vi "XYZ stage handler_MD.vi"   [LabVIEW 2012]
uses:
  <vilib>/Analysis/coordinate.llb/Euler Rotation Order.ctl
  GFG/GFGfpRefGet.vi
  GFG/GFGbooleanGet.vi
  GFG/GFGnumericGet.vi
  <vilib>/Analysis/coordinate.llb/3D Cartesian Coordinate Rotation (Euler) (Scalar).vi
  GFG/GFG library.lvlib
  <vilib>/Utility/VariantDataType/Type.ctl
  <vilib>/Utility/VariantDataType/VariantType.lvlib
  <vilib>/Analysis/NI_AALPro.lvlib
types:
  T1 = enum16{"none", "quit", "Press", "Long Press", "Long Press finished", "Short Press finished"}
  T2 = cluster{"WaveformChartRef":refnum<vi>, "DigitalRef":refnum<vi>, "ArrayRef":refnum<vi>, "TabControlRef":refnum<vi>, "EnumRef":refnum<vi>, "RingRef":refnum<vi>, "BooleanRef":refnum<vi>, "KnobRef":refnum<vi>, "SlideRef":refnum<vi>, "PathRef":refnum<vi>, "StringRef":refnum<vi>, "ComboBox":refnum<vi>, "WaveformGraphRef":refnum<vi>}
  T3 = cluster{"moveXabs":dbl, "moveYabs":dbl, "moveZabs":dbl}
  T4 = typedef "NI_AALPro.lvlib/Euler Rotation Order.ctl" = u16
  T5 = cluster{"Numeric":dbl, "Numeric":dbl, "Numeric":dbl}
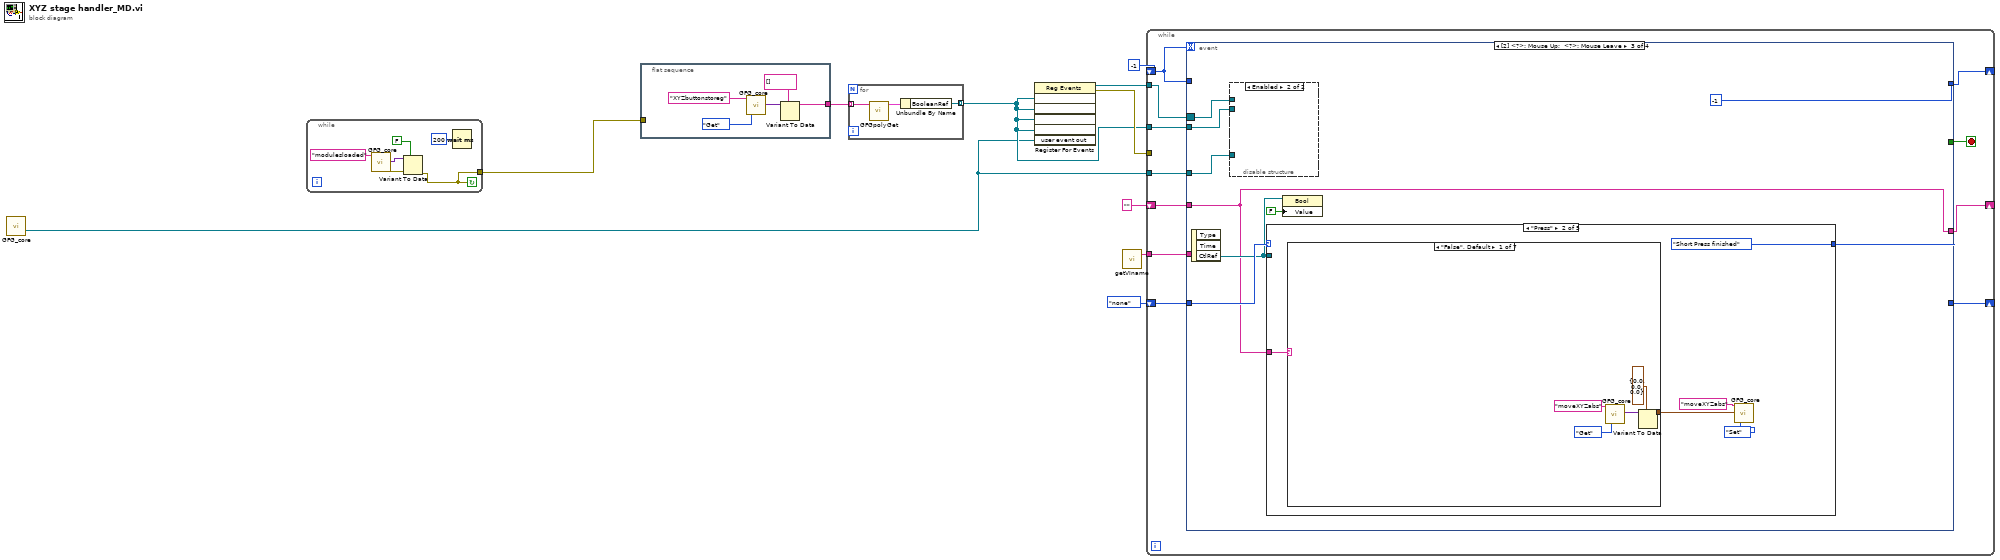
[diagram p0: block diagram]
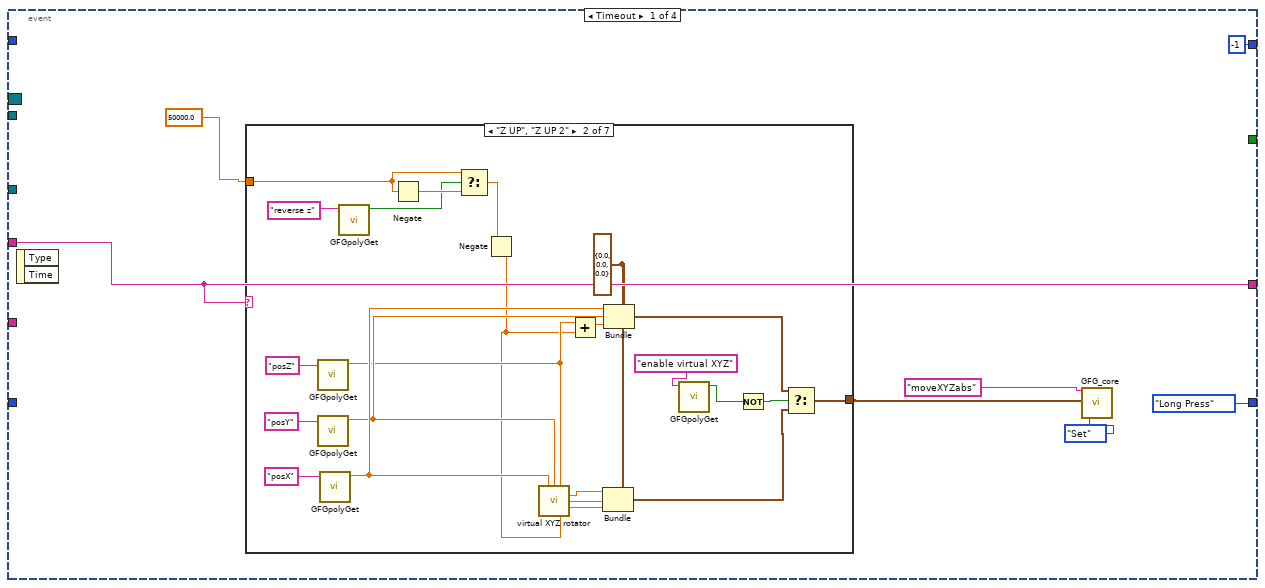
[diagram p2: hidden frame]
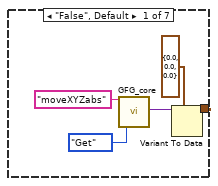
[diagram p3: hidden frame]
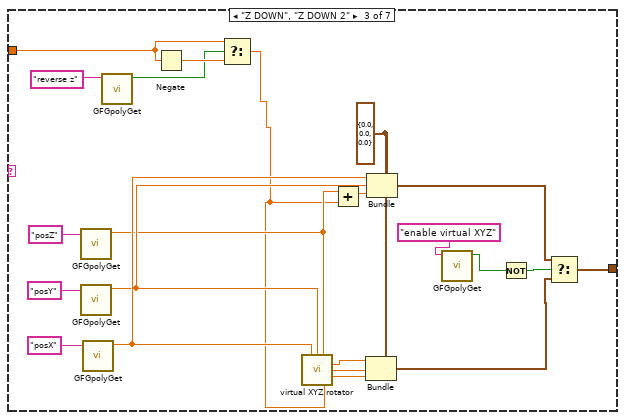
[diagram p4: hidden frame]
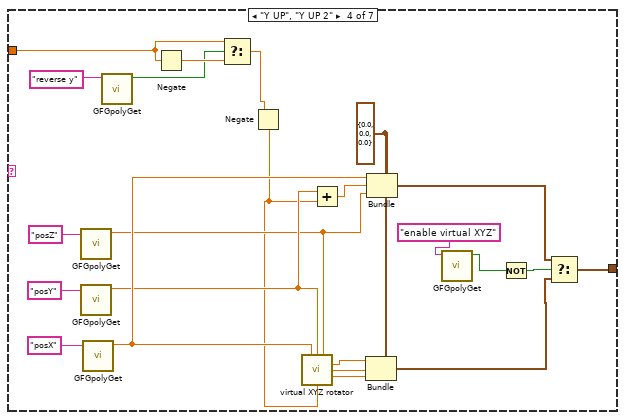
[diagram p5: hidden frame]
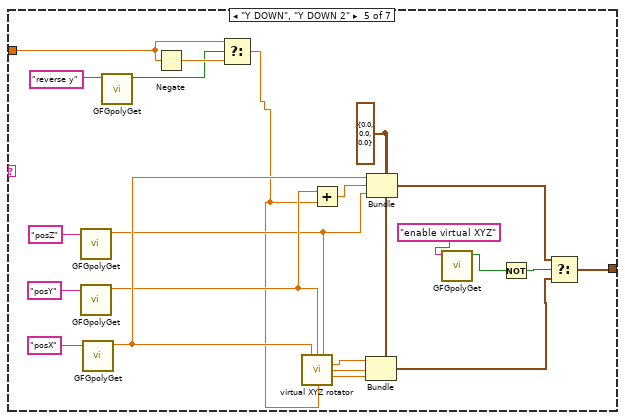
[diagram p6: hidden frame]
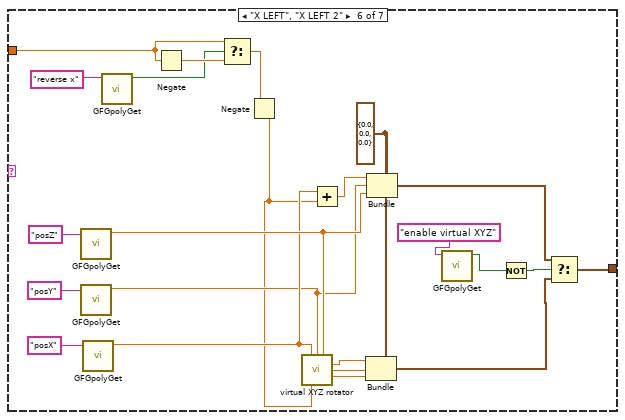
[diagram p7: hidden frame]
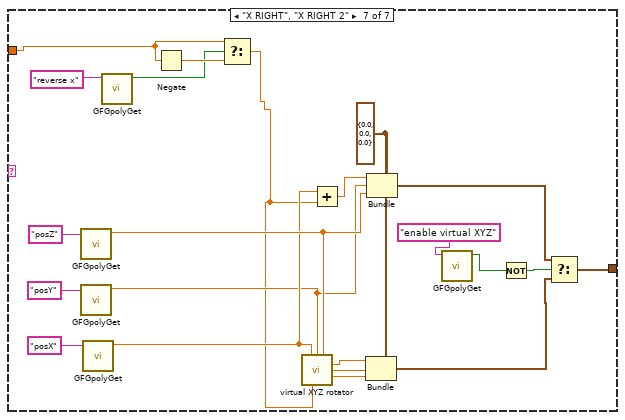
[diagram p8: hidden frame]
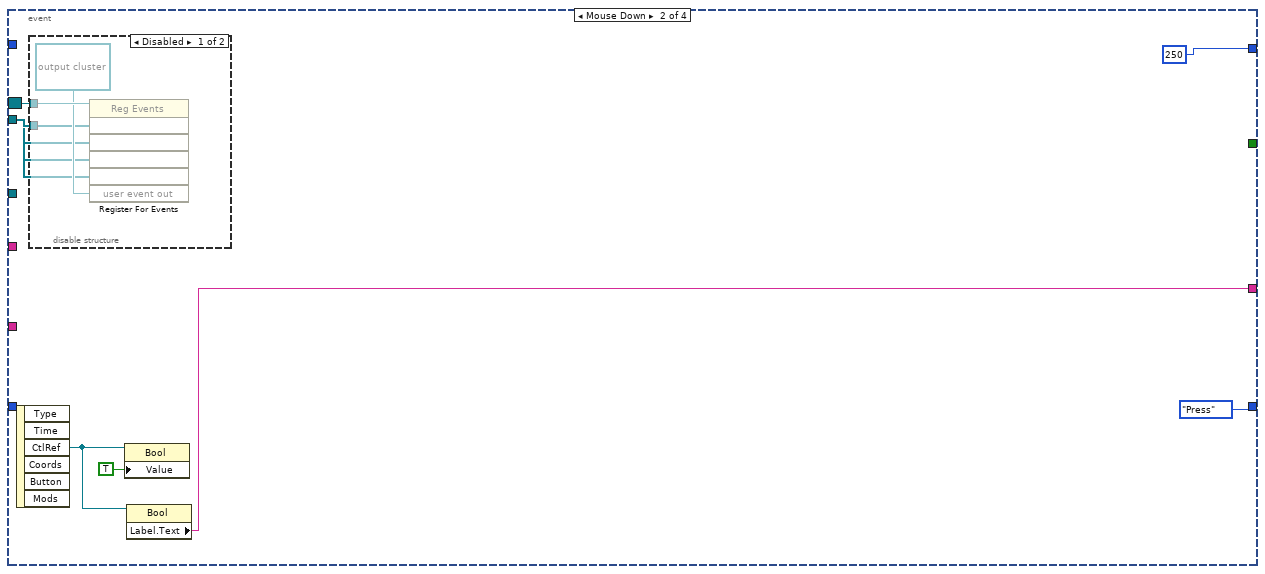
[diagram p9: hidden frame]
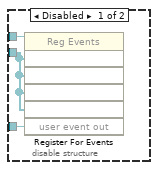
[diagram p11: hidden frame]
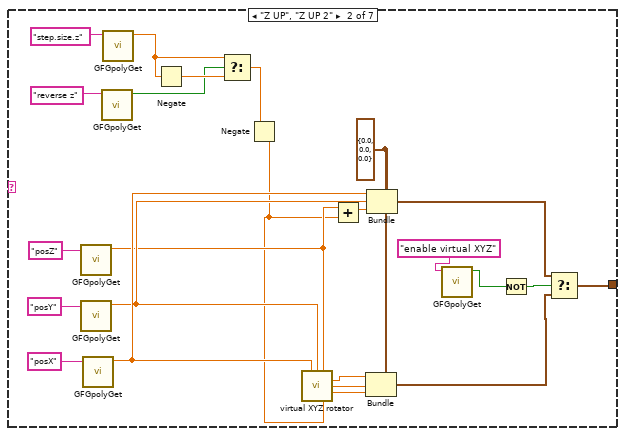
[diagram p13: hidden frame]
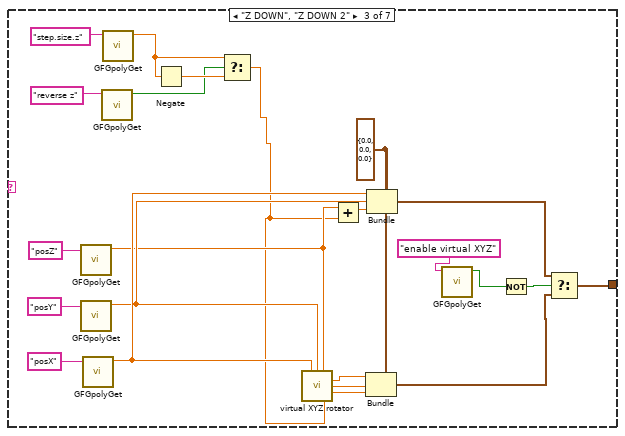
[diagram p14: hidden frame]
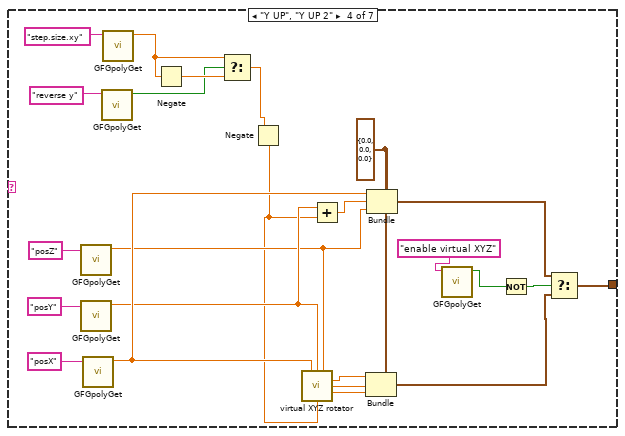
[diagram p15: hidden frame]
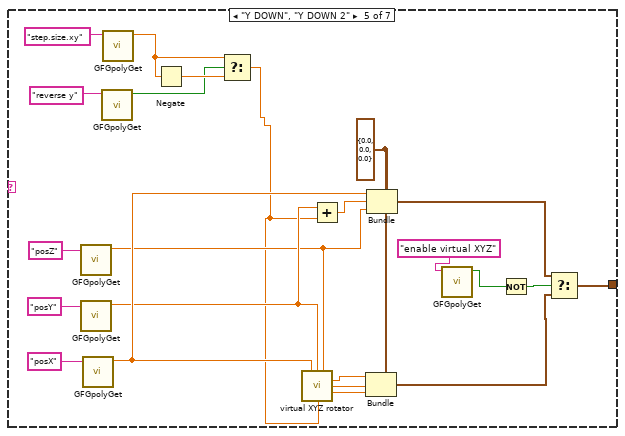
[diagram p16: hidden frame]
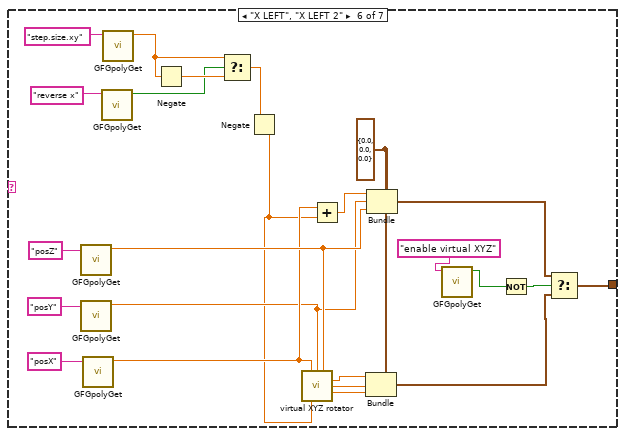
[diagram p17: hidden frame]
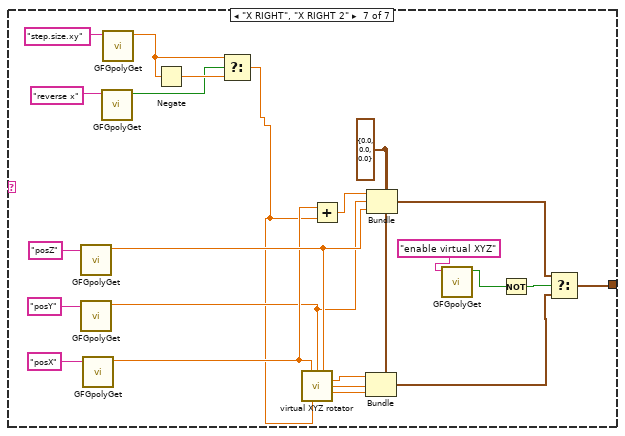
[diagram p18: hidden frame]
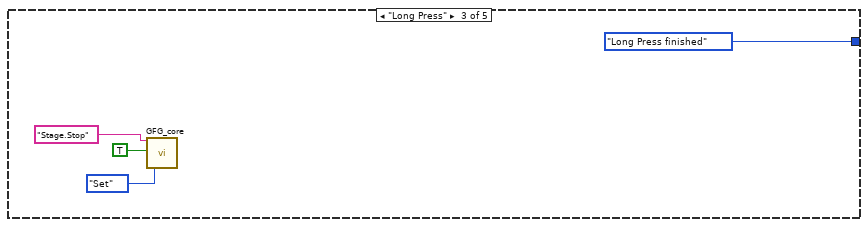
[diagram p19: hidden frame]
diagram:
  n1 = call "GFG_core.vi"() -> ("user event out"=w2:refnum<user-event>)  [unwired: 13 in, 6 out]
  n2 = while {
    tunnel: [w11] -> w1
    stop <- w11 continue-if-true
    n3 = call "GFG_core.vi"("Variable Name in"="modulesloaded") -> ("Variant Out"=w12:variant, "error out"=w14:errorcluster)  [unwired: 12 in, 5 out]
    n4 = Variant To Data(error in=w14, type=FALSE, Variant=w12) -> (error out=w11:errorcluster)  [unwired: 1 out]
    n5 = Wait (ms)(milliseconds to wait=u32 200) -> ()  [unwired: 1 out]
  }
  n6 = flat-sequence {
    tunnel: [w21] -> w3
    tunnel: w1 -> [_]
    frame #0 {
      n7 = call "GFG_core.vi"("Variable Name in"="XYZbuttonstoreg", "Action"=enum16{"Init", "Set", "Get"}."Get") -> ("Variant Out"=w17:variant)  [unwired: 11 in, 6 out]
      n8 = Variant To Data(type=string[] [], Variant=w17) -> (data=w21:string[])  [unwired: 1 in, 1 out]
    }
  }
  n9 = for {
    tunnel: w3 -> [w23] mode=indexing
    tunnel: [w22] -> w5 mode=indexing
    n10 = call-poly "GFGpolyGet.vi"("Variable Name in"=w23) -> ("output cluster"=w24:T2)  [unwired: 9 in, 1 out]
    n11 = Unbundle By Name(w24) -> ("BooleanRef"=w22:refnum<vi>)
  }
  n12 = register-events(w5, w5, w5, w5, w2) -> (reference out=w4:refnum<event-registration>, error out=w6:errorcluster)  [unwired: 2 in]
  n13 = call "getVIname.vi"() -> ("VI name"=w7:string)  [unwired: 19 in]
  n14 = while {
    shift-right: [w33] -> _
    shift-left: -1 -> [w34]
    shift-right: [w31] -> _
    shift-left: T1."none" ("Enum") -> [w32]
    shift-right: [w30] -> _
    shift-left: "" ("Label.Text") -> [w29]
    tunnel: w5 -> [w28]
    tunnel: w2 -> [w27]
    tunnel: w4 -> [w26]
    tunnel: w7 -> [w25]
    tunnel: w6 -> [_]
    stop <- w35 stop-if-true
    n15 = event shown="[2] <?>: Mouse Up;  <?>: Mouse Leave" {
      selector: w26 -> [_ w186 w195 _]
      dyn-events: _ -> [_ _ _ _]
      timeout: w34 -> [_ _ _ _]
      tunnel: [_ _ _ w375] -> w35
      tunnel: w34 -> [_ _ _ w365]
      tunnel: [-1 250 -1 w364] -> w33
      tunnel: w32 -> [_ _ w200 w374]
      tunnel: [T1."Long Press" ("Enum") T1."Press" ("Enum") w199 w374] -> w31
      tunnel: [w40 w187 w193 w371] -> w30
      tunnel: w29 -> [w40 _ w193 w371]
      tunnel: w28 -> [_ w183 w194 _]
      tunnel: w27 -> [_ _ w196 _]
      tunnel: w25 -> [_ _ _ w372]
      event Timeout {
        n16 = event-data() -> ()  [unwired: 1 in, 2 out]
        n17 = case shown="\"Z UP\", \"Z UP 2\"" w40 {
          tunnel: [w43 w53 w75 w101 w123 w147 w169] -> w36
          tunnel: 50000.0 ("-x") -> [_ w48 w71 w93 w116 w138 w161]
          frame "False", Default {
            n18 = call "GFG_core.vi"("Variable Name in"="moveXYZabs", "Action"=enum16{"Init", "Set", "Get"}."Get") -> ("Variant Out"=w45:variant)  [unwired: 11 in, 6 out]
            n19 = Variant To Data(type=T3 {"moveXabs"=0.0, "moveYabs"=0.0, "moveZabs"=0.0} ("output cluster"), Variant=w45) -> (data=w43:T3)  [unwired: 1 in, 1 out]
          }
          frame "Z UP", "Z UP 2" {
            w56 = T3 {"moveXabs"=0.0, "moveYabs"=0.0, "moveZabs"=0.0} ("output cluster")
            n20 = call-poly "GFGpolyGet.vi"("Variable Name in"="posZ") -> ("Numeric"=w60:dbl)  [unwired: 9 in, 1 out]
            n21 = call-poly "GFGpolyGet.vi"("Variable Name in"="posY") -> ("Numeric"=w61:dbl)  [unwired: 9 in, 1 out]
            n22 = call-poly "GFGpolyGet.vi"("Variable Name in"="posX") -> ("Numeric"=w62:dbl)  [unwired: 9 in, 1 out]
            n23 = call-poly "GFGpolyGet.vi"("Variable Name in"="reverse z") -> ("Boolean"=w68:bool)  [unwired: 10 in]
            n24 = Negate(x=w48) -> (-x=w69:dbl)
            n25 = Select(t=w48, s=w68, f=w69) -> (s? t:f=w50:dbl)
            n26 = Negate(x=w50) -> (-x=w49:dbl)
            n27 = call "virtual XYZ rotator.vi"("current pos X"=w62, "current pos Y"=w61, "current pos Z"=w60, "virtual Z relative"=w49) -> ("new pos X"=w59:dbl, "new pos Y"=w58:dbl, "new pos Z"=w57:dbl)  [unwired: 9 in]
            n28 = Add(x=w60, y=w49) -> (x+y=w64:dbl)
            n29 = Bundle(cluster=w56, "moveXabs"=w59, "moveYabs"=w58, "moveZabs"=w57) -> (w54:T3)
            n30 = Bundle(cluster=w56, "moveXabs"=w62, "moveYabs"=w61, "moveZabs"=w64) -> (w55:T3)
            n31 = call-poly "GFGpolyGet.vi"("Variable Name in"="enable virtual XYZ") -> ("Boolean"=w52:bool)  [unwired: 10 in]
            n32 = Not(x=w52) -> (.not. x?=w51:bool)
            n33 = Select(t=w55, s=w51, f=w54) -> (s? t:f=w53:T3)
          }
          frame "Z DOWN", "Z DOWN 2" {
            w78 = T3 {"moveXabs"=0.0, "moveYabs"=0.0, "moveZabs"=0.0} ("output cluster")
            n34 = call-poly "GFGpolyGet.vi"("Variable Name in"="posZ") -> ("Numeric"=w82:dbl)  [unwired: 9 in, 1 out]
            n35 = call-poly "GFGpolyGet.vi"("Variable Name in"="posY") -> ("Numeric"=w83:dbl)  [unwired: 9 in, 1 out]
            n36 = call-poly "GFGpolyGet.vi"("Variable Name in"="posX") -> ("Numeric"=w84:dbl)  [unwired: 9 in, 1 out]
            n37 = call-poly "GFGpolyGet.vi"("Variable Name in"="reverse z") -> ("Boolean"=w90:bool)  [unwired: 10 in]
            n38 = Negate(x=w71) -> (-x=w91:dbl)
            n39 = Select(t=w71, s=w90, f=w91) -> (s? t:f=w72:dbl)
            n40 = call "virtual XYZ rotator.vi"("current pos X"=w84, "current pos Y"=w83, "current pos Z"=w82, "virtual Z relative"=w72) -> ("new pos X"=w81:dbl, "new pos Y"=w80:dbl, "new pos Z"=w79:dbl)  [unwired: 9 in]
            n41 = Add(x=w82, y=w72) -> (x+y=w86:dbl)
            n42 = Bundle(cluster=w78, "moveXabs"=w81, "moveYabs"=w80, "moveZabs"=w79) -> (w76:T3)
            n43 = Bundle(cluster=w78, "moveXabs"=w84, "moveYabs"=w83, "moveZabs"=w86) -> (w77:T3)
            n44 = call-poly "GFGpolyGet.vi"("Variable Name in"="enable virtual XYZ") -> ("Boolean"=w74:bool)  [unwired: 10 in]
            n45 = Not(x=w74) -> (.not. x?=w73:bool)
            n46 = Select(t=w77, s=w73, f=w76) -> (s? t:f=w75:T3)
          }
          frame "Y UP", "Y UP 2" {
            w104 = T3 {"moveXabs"=0.0, "moveYabs"=0.0, "moveZabs"=0.0} ("output cluster")
            n47 = call-poly "GFGpolyGet.vi"("Variable Name in"="posZ") -> ("Numeric"=w95:dbl)  [unwired: 9 in, 1 out]
            n48 = call-poly "GFGpolyGet.vi"("Variable Name in"="posY") -> ("Numeric"=w97:dbl)  [unwired: 9 in, 1 out]
            n49 = call-poly "GFGpolyGet.vi"("Variable Name in"="posX") -> ("Numeric"=w108:dbl)  [unwired: 9 in, 1 out]
            n50 = call-poly "GFGpolyGet.vi"("Variable Name in"="reverse y") -> ("Boolean"=w113:bool)  [unwired: 10 in]
            n51 = Negate(x=w93) -> (-x=w114:dbl)
            n52 = Select(t=w93, s=w113, f=w114) -> (s? t:f=w98:dbl)
            n53 = Negate(x=w98) -> (-x=w94:dbl)
            n54 = call "virtual XYZ rotator.vi"("current pos X"=w108, "current pos Y"=w97, "current pos Z"=w95, "virtual Y relative"=w94) -> ("new pos X"=w107:dbl, "new pos Y"=w106:dbl, "new pos Z"=w105:dbl)  [unwired: 9 in]
            n55 = Add(x=w97, y=w94) -> (x+y=w96:dbl)
            n56 = Bundle(cluster=w104, "moveXabs"=w107, "moveYabs"=w106, "moveZabs"=w105) -> (w102:T3)
            n57 = Bundle(cluster=w104, "moveXabs"=w108, "moveYabs"=w96, "moveZabs"=w95) -> (w103:T3)
            n58 = call-poly "GFGpolyGet.vi"("Variable Name in"="enable virtual XYZ") -> ("Boolean"=w100:bool)  [unwired: 10 in]
            n59 = Not(x=w100) -> (.not. x?=w99:bool)
            n60 = Select(t=w103, s=w99, f=w102) -> (s? t:f=w101:T3)
          }
          frame "Y DOWN", "Y DOWN 2" {
            w126 = T3 {"moveXabs"=0.0, "moveYabs"=0.0, "moveZabs"=0.0} ("output cluster")
            n61 = call-poly "GFGpolyGet.vi"("Variable Name in"="posZ") -> ("Numeric"=w118:dbl)  [unwired: 9 in, 1 out]
            n62 = call-poly "GFGpolyGet.vi"("Variable Name in"="posY") -> ("Numeric"=w120:dbl)  [unwired: 9 in, 1 out]
            n63 = call-poly "GFGpolyGet.vi"("Variable Name in"="posX") -> ("Numeric"=w130:dbl)  [unwired: 9 in, 1 out]
            n64 = call-poly "GFGpolyGet.vi"("Variable Name in"="reverse y") -> ("Boolean"=w135:bool)  [unwired: 10 in]
            n65 = Negate(x=w116) -> (-x=w136:dbl)
            n66 = Select(t=w116, s=w135, f=w136) -> (s? t:f=w117:dbl)
            n67 = call "virtual XYZ rotator.vi"("current pos X"=w130, "current pos Y"=w120, "current pos Z"=w118, "virtual Y relative"=w117) -> ("new pos X"=w129:dbl, "new pos Y"=w128:dbl, "new pos Z"=w127:dbl)  [unwired: 9 in]
            n68 = Add(x=w120, y=w117) -> (x+y=w119:dbl)
            n69 = Bundle(cluster=w126, "moveXabs"=w129, "moveYabs"=w128, "moveZabs"=w127) -> (w124:T3)
            n70 = Bundle(cluster=w126, "moveXabs"=w130, "moveYabs"=w119, "moveZabs"=w118) -> (w125:T3)
            n71 = call-poly "GFGpolyGet.vi"("Variable Name in"="enable virtual XYZ") -> ("Boolean"=w122:bool)  [unwired: 10 in]
            n72 = Not(x=w122) -> (.not. x?=w121:bool)
            n73 = Select(t=w125, s=w121, f=w124) -> (s? t:f=w123:T3)
          }
          frame "X LEFT", "X LEFT 2" {
            w150 = T3 {"moveXabs"=0.0, "moveYabs"=0.0, "moveZabs"=0.0} ("output cluster")
            n74 = call-poly "GFGpolyGet.vi"("Variable Name in"="posZ") -> ("Numeric"=w144:dbl)  [unwired: 9 in, 1 out]
            n75 = call-poly "GFGpolyGet.vi"("Variable Name in"="posY") -> ("Numeric"=w141:dbl)  [unwired: 9 in, 1 out]
            n76 = call-poly "GFGpolyGet.vi"("Variable Name in"="posX") -> ("Numeric"=w143:dbl)  [unwired: 9 in, 1 out]
            n77 = call-poly "GFGpolyGet.vi"("Variable Name in"="reverse x") -> ("Boolean"=w158:bool)  [unwired: 10 in]
            n78 = Negate(x=w138) -> (-x=w159:dbl)
            n79 = Select(t=w138, s=w158, f=w159) -> (s? t:f=w140:dbl)
            n80 = Negate(x=w140) -> (-x=w139:dbl)
            n81 = call "virtual XYZ rotator.vi"("current pos X"=w143, "current pos Y"=w141, "current pos Z"=w144, "virtual X relative"=w139) -> ("new pos X"=w153:dbl, "new pos Y"=w152:dbl, "new pos Z"=w151:dbl)  [unwired: 9 in]
            n82 = Add(x=w143, y=w139) -> (x+y=w142:dbl)
            n83 = Bundle(cluster=w150, "moveXabs"=w153, "moveYabs"=w152, "moveZabs"=w151) -> (w148:T3)
            n84 = Bundle(cluster=w150, "moveXabs"=w142, "moveYabs"=w141, "moveZabs"=w144) -> (w149:T3)
            n85 = call-poly "GFGpolyGet.vi"("Variable Name in"="enable virtual XYZ") -> ("Boolean"=w146:bool)  [unwired: 10 in]
            n86 = Not(x=w146) -> (.not. x?=w145:bool)
            n87 = Select(t=w149, s=w145, f=w148) -> (s? t:f=w147:T3)
          }
          frame "X RIGHT", "X RIGHT 2" {
            w172 = T3 {"moveXabs"=0.0, "moveYabs"=0.0, "moveZabs"=0.0} ("output cluster")
            n88 = call-poly "GFGpolyGet.vi"("Variable Name in"="posZ") -> ("Numeric"=w166:dbl)  [unwired: 9 in, 1 out]
            n89 = call-poly "GFGpolyGet.vi"("Variable Name in"="posY") -> ("Numeric"=w163:dbl)  [unwired: 9 in, 1 out]
            n90 = call-poly "GFGpolyGet.vi"("Variable Name in"="posX") -> ("Numeric"=w165:dbl)  [unwired: 9 in, 1 out]
            n91 = call-poly "GFGpolyGet.vi"("Variable Name in"="reverse x") -> ("Boolean"=w180:bool)  [unwired: 10 in]
            n92 = Negate(x=w161) -> (-x=w181:dbl)
            n93 = Select(t=w161, s=w180, f=w181) -> (s? t:f=w162:dbl)
            n94 = call "virtual XYZ rotator.vi"("current pos X"=w165, "current pos Y"=w163, "current pos Z"=w166, "virtual X relative"=w162) -> ("new pos X"=w175:dbl, "new pos Y"=w174:dbl, "new pos Z"=w173:dbl)  [unwired: 9 in]
            n95 = Add(x=w165, y=w162) -> (x+y=w164:dbl)
            n96 = Bundle(cluster=w172, "moveXabs"=w175, "moveYabs"=w174, "moveZabs"=w173) -> (w170:T3)
            n97 = Bundle(cluster=w172, "moveXabs"=w164, "moveYabs"=w163, "moveZabs"=w166) -> (w171:T3)
            n98 = call-poly "GFGpolyGet.vi"("Variable Name in"="enable virtual XYZ") -> ("Boolean"=w168:bool)  [unwired: 10 in]
            n99 = Not(x=w168) -> (.not. x?=w167:bool)
            n100 = Select(t=w171, s=w167, f=w170) -> (s? t:f=w169:T3)
          }
        }
        n101 = call "GFG_core.vi"("Variable Name in"="moveXYZabs", "Variant in"=w36, "Action"=enum16{"Init", "Set", "Get"}."Set") -> ()  [unwired: 10 in, 7 out]
      }
      event Mouse Down {
        n102 = event-data() -> ("CtlRef"=w185:refnum<vi>)  [unwired: 1 in, 5 out]
        n103 = disable-structure shown="Disabled" {
          disable-tunnel: w186 -> [w192 _]
          disable-tunnel: w183 -> [w190 _]
          frame Disabled {
            n104 = register-events(reference=w192, w190, w190, w190, w190, refnum<user-event> refnum ("event source")) -> ()  [unwired: 1 in, 2 out]
          }
          frame Enabled {
          }
        }
        n105 = property class="Bool"(reference=w185, "Value"=TRUE) -> ()  [unwired: 1 in, 2 out]
        n106 = property class="Bool"(reference=w185) -> ("Label.Text"=w187:string)  [unwired: 1 in, 2 out]
      }
      event Mouse Up; Mouse Leave {
        n107 = event-data() -> ("CtlRef"=w198:refnum<vi>)  [unwired: 1 in, 2 out]
        n108 = disable-structure shown="Enabled" {
          disable-tunnel: w196 -> [w204 _]
          disable-tunnel: w195 -> [w203 _]
          disable-tunnel: w194 -> [w202 _]
          frame Disabled {
            n109 = register-events(reference=w203, w202, w202, w202, w202, w204) -> ()  [unwired: 1 in, 2 out]
          }
          frame Enabled {
          }
        }
        n110 = case shown="\"Press\"" w200 {
          selector: w200 -> [w205 _ _ w361 w362]
          tunnel: [w205 T1."Short Press finished" ("Enum") T1."Long Press finished" ("Enum") w361 w362] -> w199
          tunnel: w198 -> [_ _ _ _ _]
          tunnel: w193 -> [_ w209 _ _ _]
          frame "none", Default {
          }
          frame "Press" {
            n111 = case shown="\"False\", Default" w209 {
              tunnel: [w211 w220 w243 w270 w293 w318 w341] -> w206
              frame "False", Default {
                n112 = call "GFG_core.vi"("Variable Name in"="moveXYZabs", "Action"=enum16{"Init", "Set", "Get"}."Get") -> ("Variant Out"=w213:variant)  [unwired: 11 in, 6 out]
                n113 = Variant To Data(type=T3 {"moveXabs"=0.0, "moveYabs"=0.0, "moveZabs"=0.0} ("output cluster"), Variant=w213) -> (data=w211:T3)  [unwired: 1 in, 1 out]
              }
              frame "Z UP", "Z UP 2" {
                w223 = T3 {"moveXabs"=0.0, "moveYabs"=0.0, "moveZabs"=0.0} ("output cluster")
                n114 = call-poly "GFGpolyGet.vi"("Variable Name in"="posZ") -> ("Numeric"=w227:dbl)  [unwired: 9 in, 1 out]
                n115 = call-poly "GFGpolyGet.vi"("Variable Name in"="posY") -> ("Numeric"=w228:dbl)  [unwired: 9 in, 1 out]
                n116 = call-poly "GFGpolyGet.vi"("Variable Name in"="posX") -> ("Numeric"=w229:dbl)  [unwired: 9 in, 1 out]
                n117 = call-poly "GFGpolyGet.vi"("Variable Name in"="reverse z") -> ("Boolean"=w235:bool)  [unwired: 10 in]
                n118 = call-poly "GFGpolyGet.vi"("Variable Name in"="step.size.z") -> ("Numeric"=w236:dbl)  [unwired: 9 in, 1 out]
                n119 = Negate(x=w236) -> (-x=w237:dbl)
                n120 = Select(t=w236, s=w235, f=w237) -> (s? t:f=w217:dbl)
                n121 = Negate(x=w217) -> (-x=w216:dbl)
                n122 = call "virtual XYZ rotator.vi"("current pos X"=w229, "current pos Y"=w228, "current pos Z"=w227, "virtual Z relative"=w216) -> ("new pos X"=w226:dbl, "new pos Y"=w225:dbl, "new pos Z"=w224:dbl)  [unwired: 9 in]
                n123 = Add(x=w227, y=w216) -> (x+y=w231:dbl)
                n124 = Bundle(cluster=w223, "moveXabs"=w226, "moveYabs"=w225, "moveZabs"=w224) -> (w221:T3)
                n125 = Bundle(cluster=w223, "moveXabs"=w229, "moveYabs"=w228, "moveZabs"=w231) -> (w222:T3)
                n126 = call-poly "GFGpolyGet.vi"("Variable Name in"="enable virtual XYZ") -> ("Boolean"=w219:bool)  [unwired: 10 in]
                n127 = Not(x=w219) -> (.not. x?=w218:bool)
                n128 = Select(t=w222, s=w218, f=w221) -> (s? t:f=w220:T3)
              }
              frame "Z DOWN", "Z DOWN 2" {
                w246 = T3 {"moveXabs"=0.0, "moveYabs"=0.0, "moveZabs"=0.0} ("output cluster")
                n129 = call-poly "GFGpolyGet.vi"("Variable Name in"="posZ") -> ("Numeric"=w250:dbl)  [unwired: 9 in, 1 out]
                n130 = call-poly "GFGpolyGet.vi"("Variable Name in"="posY") -> ("Numeric"=w251:dbl)  [unwired: 9 in, 1 out]
                n131 = call-poly "GFGpolyGet.vi"("Variable Name in"="posX") -> ("Numeric"=w252:dbl)  [unwired: 9 in, 1 out]
                n132 = call-poly "GFGpolyGet.vi"("Variable Name in"="reverse z") -> ("Boolean"=w258:bool)  [unwired: 10 in]
                n133 = call-poly "GFGpolyGet.vi"("Variable Name in"="step.size.z") -> ("Numeric"=w259:dbl)  [unwired: 9 in, 1 out]
                n134 = Negate(x=w259) -> (-x=w260:dbl)
                n135 = Select(t=w259, s=w258, f=w260) -> (s? t:f=w240:dbl)
                n136 = call "virtual XYZ rotator.vi"("current pos X"=w252, "current pos Y"=w251, "current pos Z"=w250, "virtual Z relative"=w240) -> ("new pos X"=w249:dbl, "new pos Y"=w248:dbl, "new pos Z"=w247:dbl)  [unwired: 9 in]
                n137 = Add(x=w250, y=w240) -> (x+y=w254:dbl)
                n138 = Bundle(cluster=w246, "moveXabs"=w249, "moveYabs"=w248, "moveZabs"=w247) -> (w244:T3)
                n139 = Bundle(cluster=w246, "moveXabs"=w252, "moveYabs"=w251, "moveZabs"=w254) -> (w245:T3)
                n140 = call-poly "GFGpolyGet.vi"("Variable Name in"="enable virtual XYZ") -> ("Boolean"=w242:bool)  [unwired: 10 in]
                n141 = Not(x=w242) -> (.not. x?=w241:bool)
                n142 = Select(t=w245, s=w241, f=w244) -> (s? t:f=w243:T3)
              }
              frame "Y UP", "Y UP 2" {
                w273 = T3 {"moveXabs"=0.0, "moveYabs"=0.0, "moveZabs"=0.0} ("output cluster")
                n143 = call-poly "GFGpolyGet.vi"("Variable Name in"="posZ") -> ("Numeric"=w264:dbl)  [unwired: 9 in, 1 out]
                n144 = call-poly "GFGpolyGet.vi"("Variable Name in"="posY") -> ("Numeric"=w266:dbl)  [unwired: 9 in, 1 out]
                n145 = call-poly "GFGpolyGet.vi"("Variable Name in"="posX") -> ("Numeric"=w277:dbl)  [unwired: 9 in, 1 out]
                n146 = call-poly "GFGpolyGet.vi"("Variable Name in"="reverse y") -> ("Boolean"=w282:bool)  [unwired: 10 in]
                n147 = call-poly "GFGpolyGet.vi"("Variable Name in"="step.size.xy") -> ("Numeric"=w283:dbl)  [unwired: 9 in, 1 out]
                n148 = Negate(x=w283) -> (-x=w284:dbl)
                n149 = Select(t=w283, s=w282, f=w284) -> (s? t:f=w267:dbl)
                n150 = Negate(x=w267) -> (-x=w263:dbl)
                n151 = call "virtual XYZ rotator.vi"("current pos X"=w277, "current pos Y"=w266, "current pos Z"=w264, "virtual Y relative"=w263) -> ("new pos X"=w276:dbl, "new pos Y"=w275:dbl, "new pos Z"=w274:dbl)  [unwired: 9 in]
                n152 = Add(x=w266, y=w263) -> (x+y=w265:dbl)
                n153 = Bundle(cluster=w273, "moveXabs"=w276, "moveYabs"=w275, "moveZabs"=w274) -> (w271:T3)
                n154 = Bundle(cluster=w273, "moveXabs"=w277, "moveYabs"=w265, "moveZabs"=w264) -> (w272:T3)
                n155 = call-poly "GFGpolyGet.vi"("Variable Name in"="enable virtual XYZ") -> ("Boolean"=w269:bool)  [unwired: 10 in]
                n156 = Not(x=w269) -> (.not. x?=w268:bool)
                n157 = Select(t=w272, s=w268, f=w271) -> (s? t:f=w270:T3)
              }
              frame "Y DOWN", "Y DOWN 2" {
                w296 = T3 {"moveXabs"=0.0, "moveYabs"=0.0, "moveZabs"=0.0} ("output cluster")
                n158 = call-poly "GFGpolyGet.vi"("Variable Name in"="posZ") -> ("Numeric"=w288:dbl)  [unwired: 9 in, 1 out]
                n159 = call-poly "GFGpolyGet.vi"("Variable Name in"="posY") -> ("Numeric"=w290:dbl)  [unwired: 9 in, 1 out]
                n160 = call-poly "GFGpolyGet.vi"("Variable Name in"="posX") -> ("Numeric"=w300:dbl)  [unwired: 9 in, 1 out]
                n161 = call-poly "GFGpolyGet.vi"("Variable Name in"="reverse y") -> ("Boolean"=w305:bool)  [unwired: 10 in]
                n162 = call-poly "GFGpolyGet.vi"("Variable Name in"="step.size.xy") -> ("Numeric"=w306:dbl)  [unwired: 9 in, 1 out]
                n163 = Negate(x=w306) -> (-x=w307:dbl)
                n164 = Select(t=w306, s=w305, f=w307) -> (s? t:f=w287:dbl)
                n165 = call "virtual XYZ rotator.vi"("current pos X"=w300, "current pos Y"=w290, "current pos Z"=w288, "virtual Y relative"=w287) -> ("new pos X"=w299:dbl, "new pos Y"=w298:dbl, "new pos Z"=w297:dbl)  [unwired: 9 in]
                n166 = Add(x=w290, y=w287) -> (x+y=w289:dbl)
                n167 = Bundle(cluster=w296, "moveXabs"=w299, "moveYabs"=w298, "moveZabs"=w297) -> (w294:T3)
                n168 = Bundle(cluster=w296, "moveXabs"=w300, "moveYabs"=w289, "moveZabs"=w288) -> (w295:T3)
                n169 = call-poly "GFGpolyGet.vi"("Variable Name in"="enable virtual XYZ") -> ("Boolean"=w292:bool)  [unwired: 10 in]
                n170 = Not(x=w292) -> (.not. x?=w291:bool)
                n171 = Select(t=w295, s=w291, f=w294) -> (s? t:f=w293:T3)
              }
              frame "X LEFT", "X LEFT 2" {
                w321 = T3 {"moveXabs"=0.0, "moveYabs"=0.0, "moveZabs"=0.0} ("output cluster")
                n172 = call-poly "GFGpolyGet.vi"("Variable Name in"="posZ") -> ("Numeric"=w315:dbl)  [unwired: 9 in, 1 out]
                n173 = call-poly "GFGpolyGet.vi"("Variable Name in"="posY") -> ("Numeric"=w312:dbl)  [unwired: 9 in, 1 out]
                n174 = call-poly "GFGpolyGet.vi"("Variable Name in"="posX") -> ("Numeric"=w314:dbl)  [unwired: 9 in, 1 out]
                n175 = call-poly "GFGpolyGet.vi"("Variable Name in"="reverse x") -> ("Boolean"=w329:bool)  [unwired: 10 in]
                n176 = call-poly "GFGpolyGet.vi"("Variable Name in"="step.size.xy") -> ("Numeric"=w330:dbl)  [unwired: 9 in, 1 out]
                n177 = Negate(x=w330) -> (-x=w331:dbl)
                n178 = Select(t=w330, s=w329, f=w331) -> (s? t:f=w311:dbl)
                n179 = Negate(x=w311) -> (-x=w310:dbl)
                n180 = call "virtual XYZ rotator.vi"("current pos X"=w314, "current pos Y"=w312, "current pos Z"=w315, "virtual X relative"=w310) -> ("new pos X"=w324:dbl, "new pos Y"=w323:dbl, "new pos Z"=w322:dbl)  [unwired: 9 in]
                n181 = Add(x=w314, y=w310) -> (x+y=w313:dbl)
                n182 = Bundle(cluster=w321, "moveXabs"=w324, "moveYabs"=w323, "moveZabs"=w322) -> (w319:T3)
                n183 = Bundle(cluster=w321, "moveXabs"=w313, "moveYabs"=w312, "moveZabs"=w315) -> (w320:T3)
                n184 = call-poly "GFGpolyGet.vi"("Variable Name in"="enable virtual XYZ") -> ("Boolean"=w317:bool)  [unwired: 10 in]
                n185 = Not(x=w317) -> (.not. x?=w316:bool)
                n186 = Select(t=w320, s=w316, f=w319) -> (s? t:f=w318:T3)
              }
              frame "X RIGHT", "X RIGHT 2" {
                w344 = T3 {"moveXabs"=0.0, "moveYabs"=0.0, "moveZabs"=0.0} ("output cluster")
                n187 = call-poly "GFGpolyGet.vi"("Variable Name in"="posZ") -> ("Numeric"=w338:dbl)  [unwired: 9 in, 1 out]
                n188 = call-poly "GFGpolyGet.vi"("Variable Name in"="posY") -> ("Numeric"=w335:dbl)  [unwired: 9 in, 1 out]
                n189 = call-poly "GFGpolyGet.vi"("Variable Name in"="posX") -> ("Numeric"=w337:dbl)  [unwired: 9 in, 1 out]
                n190 = call-poly "GFGpolyGet.vi"("Variable Name in"="reverse x") -> ("Boolean"=w352:bool)  [unwired: 10 in]
                n191 = call-poly "GFGpolyGet.vi"("Variable Name in"="step.size.xy") -> ("Numeric"=w353:dbl)  [unwired: 9 in, 1 out]
                n192 = Negate(x=w353) -> (-x=w354:dbl)
                n193 = Select(t=w353, s=w352, f=w354) -> (s? t:f=w334:dbl)
                n194 = call "virtual XYZ rotator.vi"("current pos X"=w337, "current pos Y"=w335, "current pos Z"=w338, "virtual X relative"=w334) -> ("new pos X"=w347:dbl, "new pos Y"=w346:dbl, "new pos Z"=w345:dbl)  [unwired: 9 in]
                n195 = Add(x=w337, y=w334) -> (x+y=w336:dbl)
                n196 = Bundle(cluster=w344, "moveXabs"=w347, "moveYabs"=w346, "moveZabs"=w345) -> (w342:T3)
                n197 = Bundle(cluster=w344, "moveXabs"=w336, "moveYabs"=w335, "moveZabs"=w338) -> (w343:T3)
                n198 = call-poly "GFGpolyGet.vi"("Variable Name in"="enable virtual XYZ") -> ("Boolean"=w340:bool)  [unwired: 10 in]
                n199 = Not(x=w340) -> (.not. x?=w339:bool)
                n200 = Select(t=w343, s=w339, f=w342) -> (s? t:f=w341:T3)
              }
            }
            n201 = call "GFG_core.vi"("Variable Name in"="moveXYZabs", "Variant in"=w206, "Action"=enum16{"Init", "Set", "Get"}."Set") -> ()  [unwired: 10 in, 7 out]
          }
          frame "Long Press" {
            n202 = call "GFG_core.vi"("Variable Name in"="Stage.Stop", "Variant in"=TRUE, "Action"=enum16{"Init", "Set", "Get"}."Set") -> ()  [unwired: 10 in, 7 out]
          }
          frame "Long Press finished" {
          }
          frame "Short Press finished" {
          }
        }
        n203 = property class="Bool"(reference=w198, "Value"=FALSE) -> ()  [unwired: 1 in, 2 out]
      }
      event User Event {
        # "Less than timeout preset?"
        # "Time Elapsed between user events"
        n204 = event-data() -> ("Source VI"=w373:string, "Variable Name"=w376:string, "Variant"=w377:variant)  [unwired: 1 in, 4 out]
        n205 = case shown="\"enable.virtual.XYZ\", \"posX\", \"posX.2\", \"posY\", \"posY.2\", \"posZ\", \"posZ.2\"" w376 {
          selector: w376 -> [_ w379 w463 _ w479]
          tunnel: [_ _ _ w473 _] -> w375
          tunnel: w377 -> [_ w378 w462 w475 _]
          tunnel: w373 -> [_ w382 _ _ _]
          tunnel: w372 -> [_ w381 _ _ _]
          frame "False", Default {
          }
          frame "setX", "setX.2", "setY", "setY.2", "setZ", "setZ.2" {
            n206 = Not Equal?(x=w381, y=w382) -> (x != y?=w380:bool)
            n207 = case shown="True" w380 {
              tunnel: w379 -> [_ w400]
              tunnel: w378 -> [_ w399]
              frame False {
              }
              frame True {
                w389 = 0.0 ("current pos X")
                w394 = T3 {"moveXabs"=0.0, "moveYabs"=0.0, "moveZabs"=0.0} ("output cluster")
                n208 = call-poly "GFGpolyGet.vi"("Variable Name in"="setX") -> ("Numeric"=w405:dbl)  [unwired: 9 in, 1 out]
                n209 = call-poly "GFGpolyGet.vi"("Variable Name in"="setY") -> ("Numeric"=w404:dbl)  [unwired: 9 in, 1 out]
                n210 = call-poly "GFGpolyGet.vi"("Variable Name in"="setZ") -> ("Numeric"=w406:dbl)  [unwired: 9 in, 1 out]
                n211 = case shown="\"setZ\", \"setZ.2\"" w400 {
                  tunnel: w404 -> [w408 w413 w416 w422]
                  tunnel: w405 -> [w409 w410 w417 w423]
                  tunnel: w406 -> [w407 w411 w418 w421]
                  tunnel: w399 -> [_ w414 w419 w424]
                  tunnel: [w408 w413 w415 w422] -> w384
                  tunnel: [w409 w412 w417 w423] -> w385
                  tunnel: [w407 w411 w418 w420] -> w383
                  frame "False", Default {
                  }
                  frame "setX", "setX.2" {
                    n212 = Variant To Data(type=w410, Variant=w414) -> (data=w412:dbl)  [unwired: 1 in, 1 out]
                  }
                  frame "setY", "setY.2" {
                    n213 = Variant To Data(type=w416, Variant=w419) -> (data=w415:dbl)  [unwired: 1 in, 1 out]
                  }
                  frame "setZ", "setZ.2" {
                    n214 = Variant To Data(type=w421, Variant=w424) -> (data=w420:dbl)  [unwired: 1 in, 1 out]
                  }
                }
                n215 = call "virtual XYZ rotator.vi"("current pos X"=w389, "current pos Y"=w389, "current pos Z"=w389, "virtual X relative"=w385, "virtual Y relative"=w384, "virtual Z relative"=w383) -> ("new pos X"=w397:dbl, "new pos Y"=w396:dbl, "new pos Z"=w395:dbl)  [unwired: 7 in]
                n216 = Bundle(cluster=w394, "moveXabs"=w397, "moveYabs"=w396, "moveZabs"=w395) -> (w392:T3)
                n217 = Bundle(cluster=w394, "moveXabs"=w385, "moveYabs"=w384, "moveZabs"=w383) -> (w393:T3)
                n218 = call-poly "GFGpolyGet.vi"("Variable Name in"="enable virtual XYZ") -> ("Boolean"=w391:bool)  [unwired: 10 in]
                n219 = Not(x=w391) -> (.not. x?=w390:bool)
                n220 = Select(t=w393, s=w390, f=w392) -> (s? t:f=w386:T3)
                n221 = call "GFG_core.vi"("Variable Name in"="moveXYZabs", "Variant in"=w386, "Action"=enum16{"Init", "Set", "Get"}."Set") -> ()  [unwired: 10 in, 7 out]
              }
            }
          }
          frame "enable.virtual.XYZ", "posX", "posX.2", "posY", "posY.2", "posZ", "posZ.2" {
            w429 = enum16{"Init", "Set", "Get"}."Set" ("Action")
            w450 = T4 5 items=["X-Y-Z", "X-Z-Y", "Y-X-Z", "Y-Z-X", "Z-X-Y", "Z-Y-X", "X-Y-X", "X-Z-X", "Y-X-Y", "Y-Z-Y", "Z-X-Z", "Z-Y-Z"] ("rotation order")
            w464 = enum16{"Init", "Set", "Get"}."Set" ("Action")
            n222 = case shown="\"False\", Default" w463 {
              tunnel: w462 -> [_ w472]
              tunnel: [w468 w470] -> w439
              frame "False", Default {
                n223 = call-poly "GFGpolyGet.vi"("Variable Name in"="enable virtual XYZ") -> ("Boolean"=w468:bool)  [unwired: 10 in]
              }
              frame "enable.virtual.XYZ" {
                n224 = Variant To Data(type=TRUE, Variant=w472) -> (data=w470:bool)  [unwired: 1 in, 1 out]
                n225 = case shown="True" w470 {
                  frame False {
                  }
                  frame True {
                    n226 = call "set virtual Z rotation values.vi"() -> ()  [unwired: 12 in]
                  }
                }
              }
            }
            n227 = call-poly "GFGpolyGet.vi"("Variable Name in"="rot.vert") -> ("Numeric"=w454:dbl)  [unwired: 9 in, 1 out]
            n228 = call-poly "GFGpolyGet.vi"("Variable Name in"="rot.horiz") -> ("Numeric"=w453:dbl)  [unwired: 9 in, 1 out]
            n229 = Negate(x=w454) -> (-x=w456:dbl)
            n230 = Negate(x=w453) -> (-x=w455:dbl)
            n231 = Bundle(w455, w456, "phi"=0.0) -> (w458:cluster{dbl, dbl, "phi":dbl})  [unwired: 1 in]
            n232 = Not(x=w439) -> (.not. x?=w438:bool)
            n233 = call-poly "GFGpolyGet.vi"("Variable Name in"="posX") -> ("Numeric"=w448:dbl)  [unwired: 9 in, 1 out]
            n234 = call-poly "GFGpolyGet.vi"("Variable Name in"="posY") -> ("Numeric"=w447:dbl)  [unwired: 9 in, 1 out]
            n235 = call-poly "GFGpolyGet.vi"("Variable Name in"="posZ") -> ("Numeric"=w446:dbl)  [unwired: 9 in, 1 out]
            n236 = Bundle("Numeric"=w448, "Numeric"=w447, "Numeric"=w446) -> (w436:T5)  [unwired: 1 in]
            n237 = expression code="(x/180.0)*pi" "degrees to radians"(w458) -> (w449:cluster{dbl, dbl, "phi":dbl})
            n238 = Unbundle(w436) -> ("Numeric"=w445:dbl, "Numeric"=w444:dbl, "Numeric"=w443:dbl)
            n239 = call-poly <vilib>:"3D Cartesian Coordinate Rotation (Euler).vi"("rotation order"=w450, "Euler Angles"=w449, "z"=w443, "y"=w444, "x"=w445) -> ("z out"=w440:dbl, "y out"=w441:dbl, "x out"=w442:dbl)  [unwired: 3 in, 1 out]
            n240 = Bundle("x out"=w442, "y out"=w441, "z out"=w440) -> (w437:cluster{"x out":dbl, "y out":dbl, "z out":dbl})  [unwired: 1 in]
            n241 = Select(t=w436, s=w438, f=w437) -> (s? t:f=w425:cluster{"x out":dbl, "y out":dbl, "z out":dbl})
            n242 = Unbundle(w425) -> ("x out"=w435:dbl, "y out"=w434:dbl, "z out"=w433:dbl)
            n243 = Unbundle(w425) -> ("x out"=w430:dbl, "y out"=w431:dbl, "z out"=w432:dbl)
            n244 = call "GFG_core.vi"("Variable Name in"="setX", "Variant in"=w435, "Action"=w464) -> ()  [unwired: 10 in, 7 out]
            n245 = call "GFG_core.vi"("Variable Name in"="setY", "Variant in"=w434, "Action"=w464) -> ()  [unwired: 10 in, 7 out]
            n246 = call "GFG_core.vi"("Variable Name in"="setZ", "Variant in"=w433, "Action"=w464) -> ()  [unwired: 10 in, 7 out]
            n247 = call "GFG_core.vi"("Variable Name in"="setX 2", "Variant in"=w430, "Action"=w429) -> ()  [unwired: 10 in, 7 out]
            n248 = call "GFG_core.vi"("Variable Name in"="setY 2", "Variant in"=w431, "Action"=w429) -> ()  [unwired: 10 in, 7 out]
            n249 = call "GFG_core.vi"("Variable Name in"="setZ 2", "Variant in"=w432, "Action"=w429) -> ()  [unwired: 10 in, 7 out]
          }
          frame "QUIT" {
            n250 = Variant To Data(type=FALSE ("NewVal"), Variant=w475) -> (data=w473:bool)  [unwired: 1 in, 1 out]
          }
          frame "set.stage.speed" {
            n251 = call-poly "GFGpolyGet.vi"("Variable Name in"=w479) -> ("output cluster"=w478:T2)  [unwired: 9 in, 1 out]
            n252 = Unbundle By Name(w478) -> ("BooleanRef"=w477:refnum<vi>)
            n253 = call "set stage speeds.vi"() -> ()  [unwired: 12 in]
            n254 = property class="Bool"(reference=w477, "Value"=FALSE) -> ()  [unwired: 1 in, 2 out]
          }
        }
        n255 = Tick Count (ms)() -> (millisecond timer value=w370:u32)
        n256 = feedback-in #1(w370) -> ()
        n257 = feedback #1() -> (w369:u32)  [unwired: 1 in]
        n258 = Subtract(x=w370, y=w369) -> (x-y=w368:u32)
        n259 = To Long Integer(number=w368) -> (32bit integer=w363:i32)
        n260 = Less?(x=w363, y=w365) -> (x < y?=w367:bool)
        n261 = Subtract(x=w365, y=w363) -> (x-y=w366:i32)
        n262 = Select(t=w366, s=w367, f=w365) -> (s? t:f=w364:i32)
      }
    }
  }
